vi "Drive_Utils_CalculateScale.vi"(4 "Right distance":dbl, 5 "Left distance":dbl) -> (1 "Right scale":dbl=1.0, 2 "Left scale":dbl=1.0)   [LabVIEW 2009, in "Drive.lvlib" / "Drive_Utils.lvlib"]
uses:
  Drive_Utils.lvlib
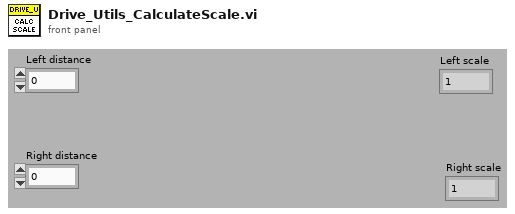
[diagram p1: front panel]
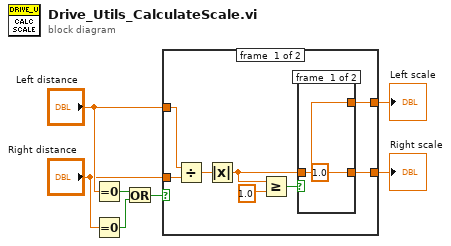
[diagram p0: block diagram]
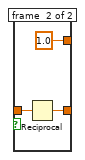
[diagram p2: hidden frame]
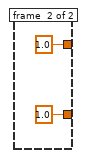
[diagram p3: hidden frame]
diagram:
  n1 = Equal To 0?(x="Left distance") -> (x = 0?=w7:bool)
  n2 = Equal To 0?(x="Right distance") -> (x = 0?=w6:bool)
  n3 = Or(x=w7, y=w6) -> (x .or. y?=w5:bool)
  n4 = case shown="False" w5 {
    tunnel: [w9 1.0 ("Left scale")] -> w4
    tunnel: [w8 1.0 ("Left scale")] -> w3
    tunnel: "Left distance" -> [w15 _]
    tunnel: "Right distance" -> [w14 _]
    frame #0 {
      n5 = Divide(x=w15, y=w14) -> (x/y=w13:dbl)
      n6 = Absolute Value(x=w13) -> (abs(x)=w10:dbl)
      n7 = Greater Or Equal?(x=w10, y=1.0) -> (x >= y?=w12:bool)
      n8 = case shown="False" w12 {
        tunnel: w10 -> [w16 w19]
        tunnel: [w16 1.0] -> w9
        tunnel: [1.0 w18] -> w8
        frame #0 {
        }
        frame #1 {
          n9 = Reciprocal(x=w19) -> (1/x=w18:dbl)
        }
      }
    }
    frame #1 {
    }
  }
  "Left scale" <- w4
  "Right scale" <- w3
